vi "4155C Config VSU.vi"(0 "VISA session":refnum<visa-resource-name>, 1 "standby":bool, 5 "unit to configure":u32(slide) max=5 scale=0.0..1.0, 9 "function":u32(slide) max=4 scale=0.0..4.0, 11 "error in (no error)":errorcluster, 12 "V name (max 6 chars)":string) -> (4 "dup VISA resource name":refnum<visa-resource-name>, 15 "error out":errorcluster)   [LabVIEW 2019]
doc: "This VI configures an SMU for SWEEP mode measurement. \n\nThis VI corresponds to the Channel Definition Page of the instrument (when Measurement Mode is SWEEP). In general, it allows every setting change that can be made via the instrument's front panel although the change may cause a setting conflict when a measurement is initialied. This VI doesnot allow (by reporting an error) setting changes that can not be made via the instrument's front panel. For example, you may not set Series Resistance for units other than SMU1, SMU2/5.\n\n** The instrument used in the development of this instrument driver does not have an Expander Unit installed. Therefore commands related to SMU5/6 have not been verified."
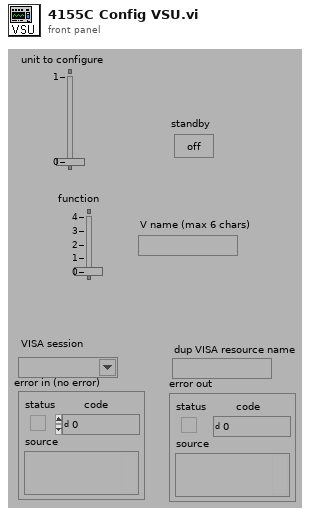
[diagram p1: front panel]
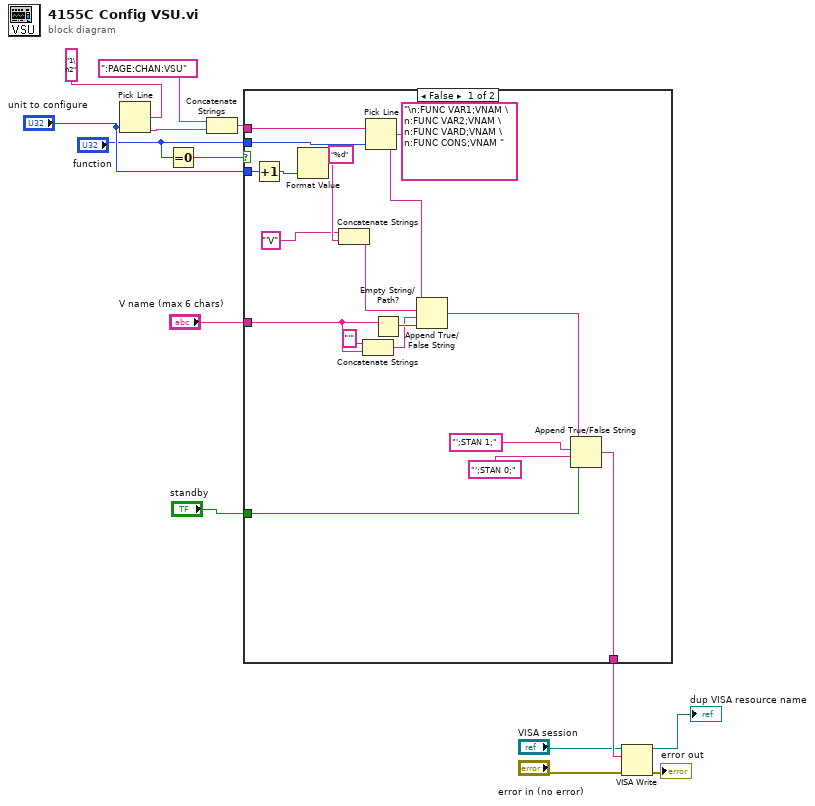
[diagram p0: block diagram]
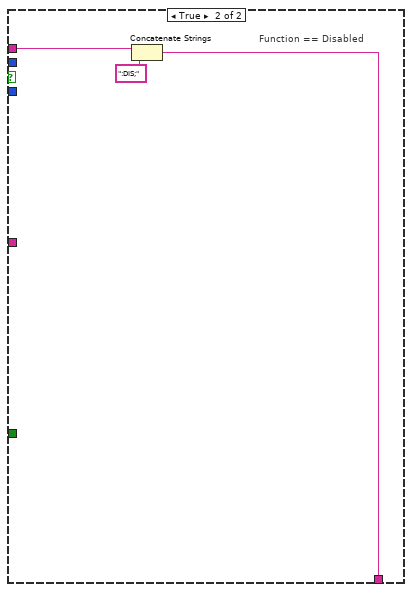
[diagram p2: hidden frame]
diagram:
  n1 = Pick Line(multi-line string="1\n2", line index="unit to configure") -> (output string=w1:string)  [unwired: 1 in]
  n2 = Equal To 0?(x="function") -> (x = 0?=w9:bool)
  n3 = Concatenate Strings(":PAGE:CHAN:VSU", w1) -> (w3:string)
  n4 = case shown="False" w9 {
    tunnel: w3 -> [w19 w36]
    tunnel: "function" -> [w32 _]
    tunnel: "unit to configure" -> [w21 _]
    tunnel: "V name (max 6 chars)" -> [w25 _]
    tunnel: "standby" -> [w16 _]
    tunnel: [w15 w34] -> w11
    frame False {
      n5 = Increment(x=w21) -> (x+1=w20:u32)
      n6 = Format Value(format string="%d", value (0)=w20) -> (output string=w30:string)  [unwired: 1 in]
      n7 = Concatenate Strings("'V", w30) -> (w28:string)
      n8 = Concatenate Strings("'", w25) -> (w24:string)
      n9 = Pick Line(string ("")=w19, multi-line string="\n:FUNC VAR1;VNAM \n:FUNC VAR2;VNAM \n:FUNC VARD;VNAM \n:FUNC CONS;VNAM ", line index=w32) -> (output string=w18:string)
      n10 = Empty String/Path?(string/path=w25) -> (empty?=w27:bool)
      n11 = Append True/False String(1:w27, 2:w24, 3:w28, 4:w18) -> (0:w17:string)
      n12 = Append True/False String(1:w16, 2:"';STAN 0;", 3:"';STAN 1;", 4:w17) -> (0:w15:string)
    }
    frame True {
      # "Function == Disabled"
      n13 = Concatenate Strings(w36, ":DIS;") -> (w34:string)
    }
  }
  n14 = VISA Write(VISA resource name="VISA session", write buffer=w11, error in (no error)="error in (no error)") -> (VISA resource name out=→"dup VISA resource name":refnum<visa-resource-name>, error out=→"error out":errorcluster)  [unwired: 1 out]
